vi "Reduce Variance.vi"(11 "Array Data":string[][](array[string])) -> (3 "Least Variable Data":string[][](array[string]))   [LabVIEW 2020]
uses:
  <vilib>/Analysis/NI_AALBase.lvlib
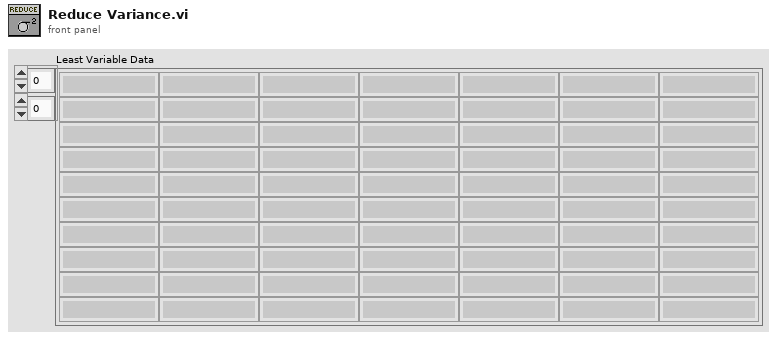
[diagram p1: front panel]
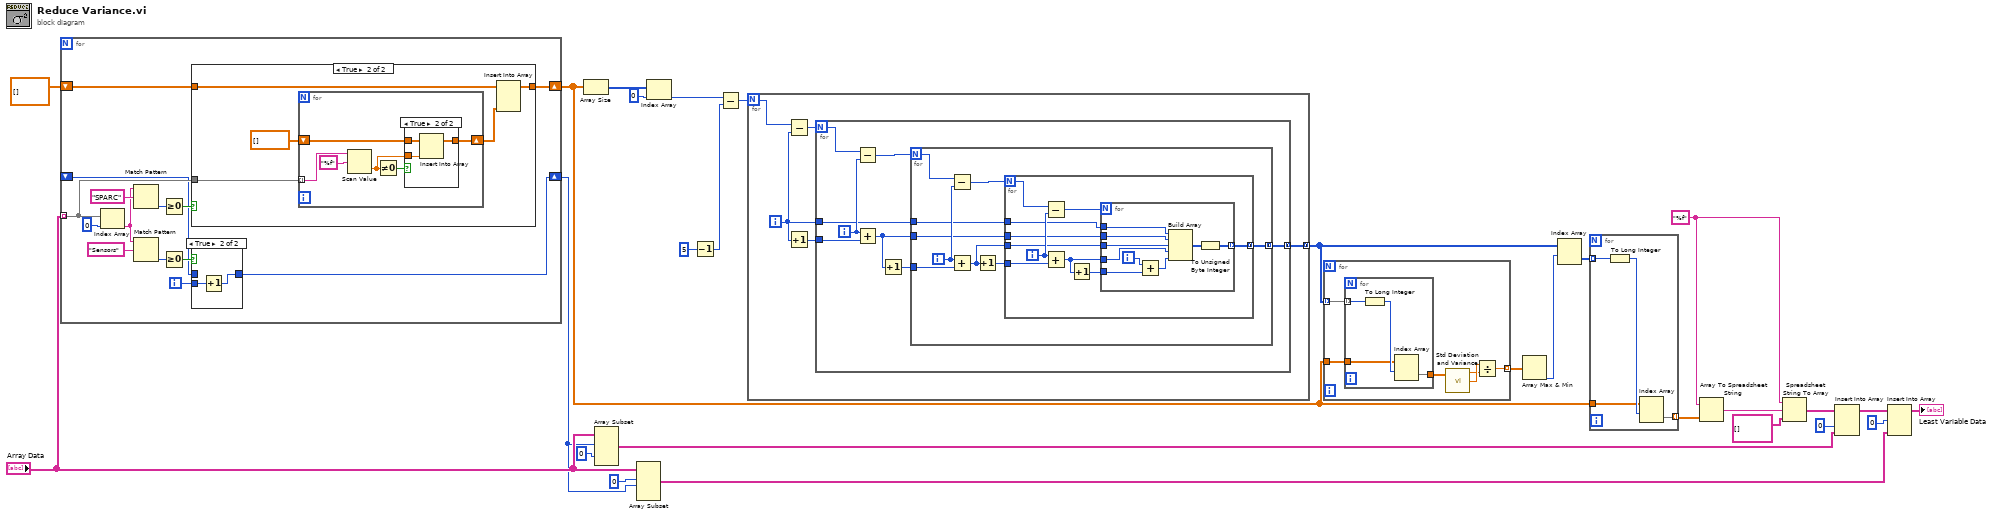
[diagram p0: block diagram]
diagram:
  w9 = "%f" ("format string")
  n1 = for {
    tunnel: "Array Data" -> [w41] mode=indexing
    shift-right: [w36] -> w17
    shift-left: dbl[][] [] ("Array") -> [w37]
    shift-right: [w29] -> w6
    shift-left: _ -> [w28]
    i -> [w30]
    n2 = Index Array(array=w41, index=0) -> (element=w33:string)
    n3 = Match Pattern(string=w33, regular expression="SPARC" ("element")) -> (offset past match=w39:i32)  [unwired: 1 in, 3 out]
    n4 = Match Pattern(string=w33, regular expression="Sensors") -> (offset past match=w34:i32)  [unwired: 1 in, 3 out]
    n5 = Greater Or Equal To 0?(x=w39) -> (x >= 0?=w35:bool)
    n6 = Greater Or Equal To 0?(x=w34) -> (x >= 0?=w31:bool)
    n7 = case shown="True" w35 {
      tunnel: w41 -> [_ w49]
      tunnel: w37 -> [w45 w48]
      tunnel: [w45 w46] -> w36
      frame False {
      }
      frame True {
        n8 = for {
          tunnel: w49 -> [w55] mode=indexing
          shift-right: [w52] -> w47
          shift-left: dbl[] [] -> [w53]
          n9 = Scan Value(string=w55, format string="%f") -> (value=w54:dbl)  [unwired: 1 in, 1 out]
          n10 = Not Equal To 0?(x=w54) -> (x != 0?=w51:bool)
          n11 = case shown="True" w51 {
            tunnel: w54 -> [_ w60]
            tunnel: w53 -> [w57 w59]
            tunnel: [w57 w58] -> w52
            frame False {
            }
            frame True {
              n12 = Insert Into Array(array=w59, new element=w60) -> (w58:dbl[])  [unwired: 1 in]
            }
          }
        }
        n13 = Insert Into Array(array=w48, new element=w47) -> (w46:dbl[][])  [unwired: 2 in]
      }
    }
    n14 = case shown="True" w31 {
      tunnel: w30 -> [_ w44]
      tunnel: [w42 w43] -> w29
      tunnel: w28 -> [w42 _]
      frame False {
      }
      frame True {
        n15 = Increment(x=w44) -> (x+1=w43:i32)
      }
    }
  }
  n16 = Array Size(array=w17) -> (size(s)=w26:i32[])
  n17 = Array Subset(array="Array Data", index (row)=w6, index (col)=0 ("index")) -> (w5:string[][])  [unwired: 2 in]
  n18 = Array Subset(array="Array Data", index (row)=0 ("index"), length (row)=w6) -> (w10:string[][])  [unwired: 2 in]
  n19 = Index Array(array=w26, index=0) -> (element=w21:i32)
  n20 = Decrement(x=5) -> (x-1=w22:i32)
  n21 = Subtract(x=w21, y=w22) -> (x-y=w24:i32)
  n22 = for {
    N: w24 -> [w64]
    tunnel: [w65] -> w19 mode=concatenating
    i -> [w61]
    n23 = Subtract(x=w64, y=w61) -> (x-y=w63:i32)
    n24 = Increment(x=w61) -> (x+1=w62:i32)
    n25 = for {
      N: w63 -> [w72]
      tunnel: [w73] -> w65 mode=concatenating
      tunnel: w62 -> [w70]
      tunnel: w61 -> [w68]
      i -> [w71]
      n26 = Subtract(x=w72, y=w71) -> (x-y=w66:i32)
      n27 = Add(x=w71, y=w70) -> (x+y=w67:i32)
      n28 = Increment(x=w67) -> (x+1=w69:i32)
      n29 = for {
        N: w66 -> [w81]
        tunnel: [w82] -> w73 mode=concatenating
        tunnel: w69 -> [w80]
        tunnel: w68 -> [w76]
        tunnel: w67 -> [w75]
        i -> [w79]
        n30 = Subtract(x=w81, y=w79) -> (x-y=w78:i32)
        n31 = Add(x=w79, y=w80) -> (x+y=w74:i32)
        n32 = Increment(x=w74) -> (x+1=w77:i32)
        n33 = for {
          N: w78 -> [w90]
          tunnel: [w91] -> w82 mode=concatenating
          tunnel: w77 -> [w88]
          tunnel: w76 -> [w86]
          tunnel: w75 -> [w85]
          tunnel: w74 -> [w84]
          i -> [w87]
          n34 = Subtract(x=w90, y=w87) -> (x-y=w89:i32)
          n35 = Add(x=w87, y=w88) -> (x+y=w83:i32)
          n36 = Increment(x=w83) -> (x+1=w92:i32)
          n37 = for {
            N: w89 -> [_]
            tunnel: w92 -> [w100]
            tunnel: [w99] -> w91 mode=indexing
            tunnel: w86 -> [w97]
            tunnel: w85 -> [w96]
            tunnel: w84 -> [w95]
            tunnel: w83 -> [w94]
            i -> [w101]
            n38 = Add(x=w101, y=w100) -> (x+y=w98:i32)
            n39 = Build Array(w97, w96, w95, w94, w98) -> (w93:i32[])
            n40 = To Unsigned Byte Integer(number=w93) -> (unsigned 8bit integer=w99:u8[])
          }
        }
      }
    }
  }
  n41 = for {
    tunnel: w19 -> [w107] mode=indexing
    tunnel: w17 -> [w106]
    tunnel: [w102] -> w20 mode=indexing
    n42 = for {
      tunnel: w107 -> [w110] mode=indexing
      tunnel: w106 -> [w109]
      tunnel: [w108] -> w105
      n43 = To Long Integer(number=w110) -> (32bit integer=w111:i32)
      n44 = Index Array(array=w109, index (row)=w111) -> (element=w108:dbl[])  [unwired: 1 in]
    }
    n45 = call <vilib>:"Std Deviation and Variance.vi"("X"=w105) -> ("mean"=w103:dbl, "standard deviation"=w104:dbl)  [unwired: 1 in, 1 out]
    n46 = Divide(x=w104, y=w103) -> (x/y=w102:dbl)
  }
  n47 = Array Max & Min(array=w20) -> (min index (indices)=w18:i32)  [unwired: 3 out]
  n48 = Index Array(array=w19, index (row)=w18) -> (element=w16:u8[])  [unwired: 1 in]
  n49 = for {
    tunnel: w16 -> [w114] mode=indexing
    tunnel: w17 -> [w113]
    tunnel: [w112] -> w15 mode=indexing
    n50 = To Long Integer(number=w114) -> (32bit integer=w115:i32)
    n51 = Index Array(array=w113, index (row)=w115) -> (element=w112:dbl[])  [unwired: 1 in]
  }
  n52 = Array To Spreadsheet String(array=w15, 3:w9) -> (spreadsheet string=w13:string)  [unwired: 1 in]
  n53 = Spreadsheet String To Array(format string=w9, spreadsheet string=w13, array type (2D Dbl)=string[][] []) -> (array=w3:string[][])  [unwired: 1 in]
  n54 = Insert Into Array(array=w3, index (col)=0 ("disabled index (col)"), new element=w5) -> (w1:string[][])  [unwired: 1 in]
  n55 = Insert Into Array(array=w1, index (row)=0, new element=w10) -> (→"Least Variable Data":string[][])  [unwired: 1 in]
